vi "Credit update1.vi"(8 "error in (no error)":errorcluster, 10 "Credit":dbl, 11 "UI Actor in":refnum<class "UI Actor.lvclass">) -> (0 "error out":errorcluster, 3 "UI Actor out":refnum<class "UI Actor.lvclass">)   [LabVIEW 2019, in "UI Actor.lvlib" / "UI Actor.lvclass"]
uses:
  UI Actor.lvclass
  UI Actor.lvclass/UI Actor.ctl
  Actor M Messages/Update M Msg/Update M Msg.lvclass/Update M Msg.ctl
  <vilib>/ActorFramework/Message Enqueuer/Message Enqueuer.lvclass/Message Enqueuer.ctl
  <vilib>/ActorFramework/Message Enqueuer/Enqueue.vi
  Actor M Messages/Update M Msg/Update M Msg.lvclass
  C:/Program Files (x86)/National Instruments/LabVIEW 2019/vi.lib/ActorFramework/Message/Message.lvclass
  <vilib>/ActorFramework/Message Priority Queue/Priority Enqueue.vi
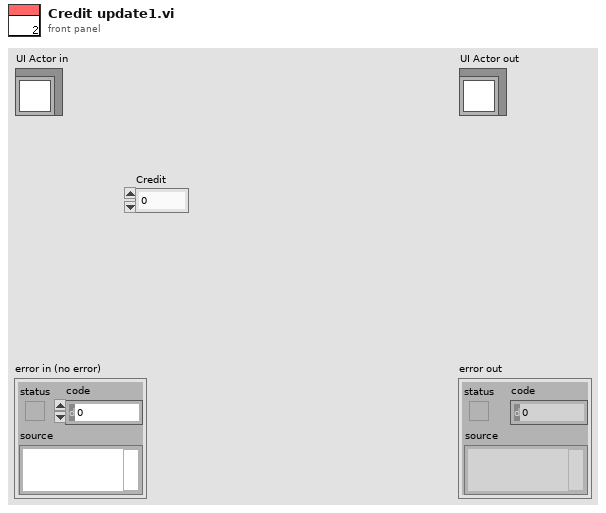
[diagram p1: front panel]
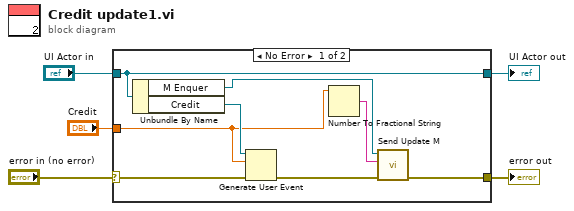
[diagram p0: block diagram]
diagram:
  n1 = case shown="No Error" "error in (no error)" {
    selector: "error in (no error)" -> [w11 w15]
    tunnel: [w6 w15] -> w4
    tunnel: [w13 w14] -> w2
    tunnel: "UI Actor in" -> [w13 w14]
    tunnel: "Credit" -> [w9 _]
    frame No Error {
      n2 = Unbundle By Name(w13) -> ("M Enquer"=w10:refnum<class "Message Enqueuer.lvclass">, "Credit"=w12:refnum<user-event>)
      n3 = Generate User Event(user event=w12, event data cluster=w9, error in=w11) -> (error out=w7:errorcluster)  [unwired: 1 in, 1 out]
      n4 = Number To Fractional String(number=w9) -> (F-format string=w8:string)  [unwired: 3 in]
      n5 = call "Send Update M.vi"("error in (no error)"=w7, "Update M"=w8, "Message Enqueuer"=w10) -> ("error out"=w6:errorcluster)  [unwired: 7 in, 1 out]
    }
    frame Error {
    }
  }
  "error out" <- w4
  "UI Actor out" <- w2
